vi "State Machine - Example.vi"() -> ()   [LabVIEW 2013, in "State Machine.lvlib"]
uses:
  State Machine.lvlib
panel:
  in  "Inject":bool
  out "timed out? 2":bool
  out "timed out?":bool
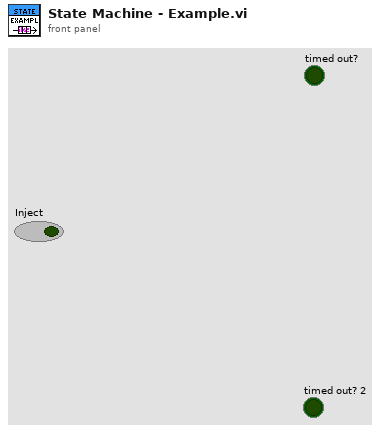
[diagram p1: front panel]
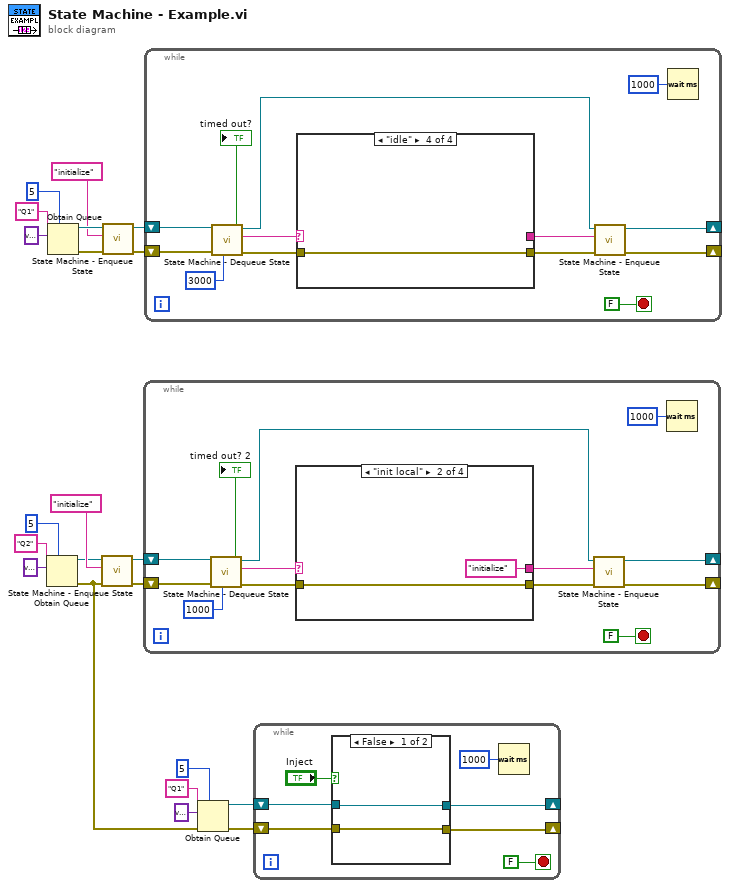
[diagram p0: block diagram]
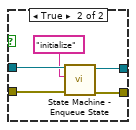
[diagram p2: hidden frame]
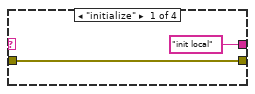
[diagram p3: hidden frame]
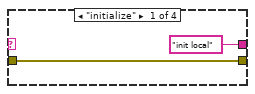
[diagram p6: hidden frame]
diagram:
  n1 = Obtain Queue(max queue size (-1, unlimited)=5, name (unnamed)="Q2", element data type=variant) -> (queue out=w10:refnum<queue>, error out=w3:errorcluster)  [unwired: 2 in, 1 out]
  n2 = Obtain Queue(max queue size (-1, unlimited)=5, name (unnamed)="Q1", element data type=variant) -> (queue out=w17:refnum<queue>, error out=w18:errorcluster)  [unwired: 2 in, 1 out]
  n3 = call "State Machine - Enqueue State.vi"("error in (no error)"=w3, "State"="initialize", "Queue In"=w10) -> ("error out"=w13:errorcluster, "Queue Out"=w12:refnum<queue>)  [unwired: 7 in]
  n4 = call "State Machine - Enqueue State.vi"("error in (no error)"=w18, "State"="initialize", "Queue In"=w17) -> ("error out"=w14:errorcluster, "Queue Out"=w15:refnum<queue>)  [unwired: 7 in]
  n5 = while {
    shift-right: [w29] -> _
    shift-left: w12 -> [w33]
    shift-right: [w28] -> _
    shift-left: w13 -> [w34]
    stop <- FALSE stop-if-true
    n6 = call "State Machine - Dequeue State.vi"("Timeout"=1000, "error in (no error)"=w34, "Queue In"=w33) -> ("error out"=w32:errorcluster, "State"=w31:string, "Queue Out"=w30:refnum<queue>, "timed out?"=→"timed out? 2":bool)  [unwired: 4 in, 1 out]
    n7 = case shown="\"init local\"" w31 {
      tunnel: w32 -> [w36 w38 w39 w40]
      tunnel: [w36 w38 w39 w40] -> w27
      tunnel: ["init local" ("State") "initialize" ("State") _ _] -> w26
      frame "initialize" {
      }
      frame "init local" {
      }
      frame Default {
      }
      frame "idle" {
      }
    }
    n8 = call "State Machine - Enqueue State.vi"("error in (no error)"=w27, "State"=w26, "Queue In"=w30) -> ("error out"=w28:errorcluster, "Queue Out"=w29:refnum<queue>)  [unwired: 7 in]
    n9 = Wait (ms)(milliseconds to wait=u32 1000) -> ()  [unwired: 1 out]
  }
  n10 = while {
    shift-right: [w48] -> _
    shift-left: w15 -> [w52]
    shift-right: [w47] -> _
    shift-left: w14 -> [w53]
    stop <- FALSE stop-if-true
    n11 = call "State Machine - Dequeue State.vi"("Timeout"=3000, "error in (no error)"=w53, "Queue In"=w52) -> ("error out"=w51:errorcluster, "State"=w50:string, "Queue Out"=w49:refnum<queue>, "timed out?"=→"timed out?":bool)  [unwired: 4 in, 1 out]
    n12 = case shown="\"idle\"" w50 {
      tunnel: w51 -> [w55 w56 w57 w58]
      tunnel: [w55 w56 w57 w58] -> w46
      tunnel: ["init local" ("State") _ _ _] -> w45
      frame "initialize" {
      }
      frame "init local" {
      }
      frame Default {
      }
      frame "idle" {
      }
    }
    n13 = call "State Machine - Enqueue State.vi"("error in (no error)"=w46, "State"=w45, "Queue In"=w49) -> ("error out"=w47:errorcluster, "Queue Out"=w48:refnum<queue>)  [unwired: 7 in]
    n14 = Wait (ms)(milliseconds to wait=u32 1000) -> ()  [unwired: 1 out]
  }
  n15 = Obtain Queue(max queue size (-1, unlimited)=5, name (unnamed)="Q1", element data type=variant, error in (no error)=w3) -> (queue out=w2:refnum<queue>, error out=w1:errorcluster)  [unwired: 1 in, 1 out]
  n16 = while {
    shift-right: [w62] -> _
    shift-left: w2 -> [w63]
    shift-right: [w60] -> _
    shift-left: w1 -> [w61]
    stop <- FALSE stop-if-true
    n17 = case shown="False" "Inject" {
      tunnel: w63 -> [w66 w72]
      tunnel: [w66 w71] -> w62
      tunnel: w61 -> [w67 w70]
      tunnel: [w67 w69] -> w60
      frame False {
      }
      frame True {
        n18 = call "State Machine - Enqueue State.vi"("error in (no error)"=w70, "State"="initialize", "Queue In"=w72) -> ("error out"=w69:errorcluster, "Queue Out"=w71:refnum<queue>)  [unwired: 7 in]
      }
    }
    n19 = Wait (ms)(milliseconds to wait=u32 1000) -> ()  [unwired: 1 out]
  }
